vi "RS232 set speed.vi"(1 "Vi steps":i32=800, 2 "Vi":i32=1000, 3 "Speed":i32(slide)=3111 min=25 max=8000 step=25 scale=25.0..8000.0) -> (0 "Command":string)   [LabVIEW 2018]
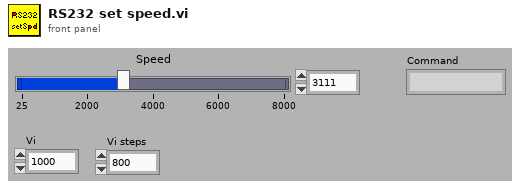
[diagram p1: front panel]
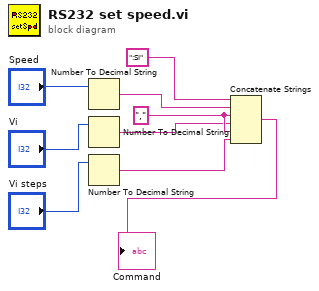
[diagram p0: block diagram]
diagram:
  w7 = ","
  n1 = Number To Decimal String(number="Speed") -> (decimal integer string=w3:string)  [unwired: 1 in]
  n2 = Number To Decimal String(number="Vi") -> (decimal integer string=w6:string)  [unwired: 1 in]
  n3 = Number To Decimal String(number="Vi steps") -> (decimal integer string=w8:string)  [unwired: 1 in]
  n4 = Concatenate Strings(":SI", w3, w7, w6, w7, w8) -> (→"Command":string)
